vi "Sea-Level SWI Open Device.vi"(8 "error in (no error)":errorcluster, 11 "Card Number":i32) -> (0 "error out":errorcluster, 3 "Handle Out":i32, 4 "Error Code":T1)   [LabVIEW 2011]
uses:
  TypeDefs/Sea-Level SWI Error Code.ctl
  SeaIo32.dll
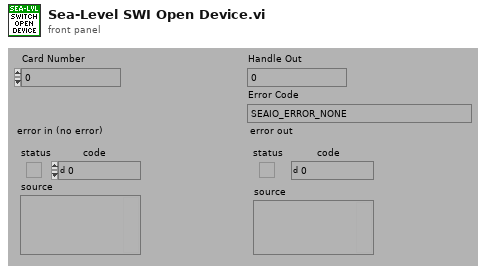
[diagram p1: front panel]
types:
  T1 = typedef "Sea-Level SWI Error Code.ctl" = enum16{"SEAIO_ERROR_NONE", "SEAIO_ERROR_PARAM", "SEAIO_ERROR_NOT_SUPPORTED", "SEAIO_ERROR_PORT_NOT_OPEN", "SEAIO_ERROR_INVALID_NAME", "SEAIO_ERROR_SHARING_VIOLATION", "SEAIO_ERROR_DRIVER_TYPE", "SEAIO_ERROR_BUFFER", "SEAIO_ERROR_INCOMPLETE", "SEAIO_ERROR_GENERAL", "SEAIO_ERROR_IO_PENDING", "SEAIO_ERROR_NO_TXBUFFER", "SEAIO_ERROR_INVALID_DEVICE_REQUEST", "SEAIO_ERROR_INVALID_HANDLE", "SEAIO_ERROR_CANCELED", "SEAIO_ERROR_LAST", "SEAIO_ERROR_NO_MEMORY", "SEAIO_ERROR_BUSY"}
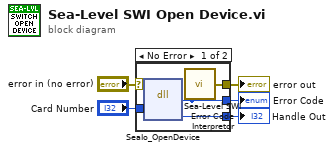
[diagram p0: block diagram]
diagram:
  n1 = case shown="No Error" "error in (no error)" {
    selector: "error in (no error)" -> [_ w10]
    tunnel: [w8 _] -> w2
    tunnel: [w9 w10] -> w3
    tunnel: "Card Number" -> [w7 _]
    tunnel: [w6 _] -> w1
    frame No Error {
      n2 = dll-call lib="C:/Development/Spartan/www/drivers/SWI/Sea-Level/SeaIo32.dll" fn="SeaIo_OpenDevice"("Card Number"=w7) -> ("Error Code"=w8:i32, "Handle"=w6:i32)  [unwired: 4 in, 3 out]
      n3 = call "Sea-Level SWI Error Code Interpretor.vi"("Error Code"=w8) -> ("error out"=w9:errorcluster)
    }
    frame Error {
    }
  }
  "Error Code" <- w2
  "Handle Out" <- w1
  "error out" <- w3
